vi "[Template]_Write.vi"(8 "error in (no error)":errorcluster, 9 "Data":T1, 11 "Tag Name":string) -> (0 "error out":errorcluster)   [LabVIEW 2010]
doc: "This VI will write the data associated with a single tag. This VI will always look up the tag index if the name changes, or if index lookup failed previously (resulting in an error). This combines the functionality of the CVT2 VIs for writes and static writes."
uses:
  [Template]_Datatype.ctl
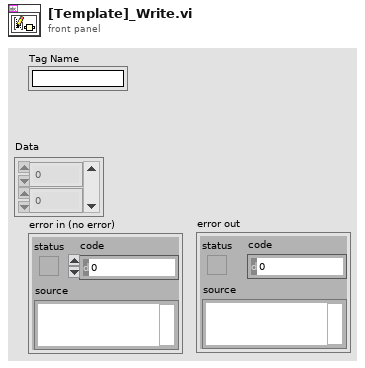
[diagram p1: front panel]
types:
  T1 = typedef "[Template]_Datatype.ctl" = i32[]
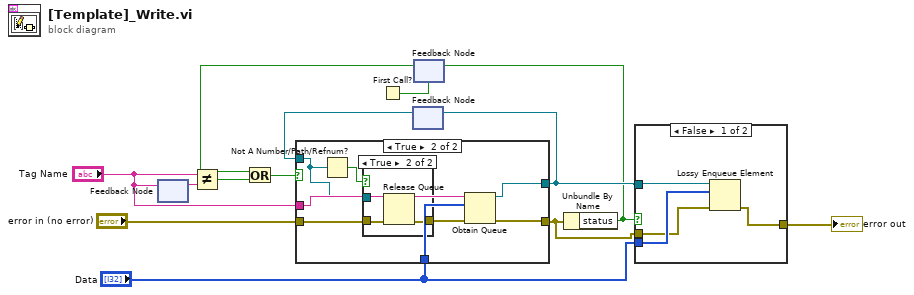
[diagram p0: block diagram]
diagram:
  n1 = feedback #1() -> (w11:string)  [unwired: 1 in]
  n2 = feedback-in #1("Tag Name") -> ()
  n3 = Not Equal?(x="Tag Name", y=w11) -> (x != y?=w5:bool)
  n4 = First Call?() -> (First Call?: T/F=w4:bool)
  n5 = feedback #2() -> (w10:refnum<queue>)  [unwired: 1 in]
  n6 = feedback #3(w4) -> (w7:bool)
  n7 = Or(x=w7, y=w5) -> (x .or. y?=w6:bool)
  n8 = case shown="True" w6 {
    tunnel: [w15 w23] -> w2
    tunnel: "error in (no error)" -> [w15 w18]
    tunnel: [w14 w20] -> w13
    tunnel: w10 -> [w14 w16]
    tunnel: "Tag Name" -> [_ w22]
    tunnel: "Data" -> [_ w21]
    frame False {
    }
    frame True {
      n9 = Not A Number/Path/Refnum?(number/path/refnum=w16) -> (NaN/Path/Refnum?=w19:bool)
      n10 = case shown="True" w19 {
        tunnel: w18 -> [w24 w26]
        tunnel: [w24 w27] -> w17
        tunnel: w16 -> [_ w25]
        frame False {
        }
        frame True {
          n11 = Release Queue(queue=w25, error in (no error)=w26) -> (error out=w27:errorcluster)  [unwired: 1 in, 2 out]
        }
      }
      n12 = Obtain Queue(name (unnamed)=w22, element data type=w21, error in (no error)=w17) -> (queue out=w20:refnum<queue>, error out=w23:errorcluster)  [unwired: 2 in, 1 out]
    }
  }
  n13 = feedback-in #2(w13) -> ()
  n14 = Unbundle By Name(w2) -> ("status"=w8:bool)
  n15 = feedback-in #3(w8) -> ()
  n16 = case shown="False" w8 {
    tunnel: w13 -> [w31 _]
    tunnel: "Data" -> [w30 _]
    tunnel: w2 -> [w29 w32]
    tunnel: [w28 w32] -> w1
    frame False {
      n17 = Lossy Enqueue Element(queue=w31, element=w30, error in (no error)=w29) -> (error out=w28:errorcluster)  [unwired: 3 out]
    }
    frame True {
    }
  }
  "error out" <- w1
